vi "Write Power FIFO Direct Dispatch.vi"(6 "FIFO Timestamps":T2, 8 "error in (no error)":errorcluster, 9 "Timeout (ms)":i32=100, 10 "Power Waveform In":T1, 11 "CIFTag in":refnum<class "CIFChannels.lvclass">) -> (0 "error out":errorcluster, 1 "timed out?":bool, 2 "Power Waveform Out":T1, 3 "CIFTag out":refnum<class "CIF_NIChn_Fifo_Power_DVR.lvclass">)   [LabVIEW 2021, in "CIF_NIChn_Fifo_Power_DVR.lvclass"]
uses:
  CIF_NIChn_Fifo_Power_DVR.lvclass
  D:/dev/CIF-LVCore/src/Channels/CIFChannels/CIFChannels.lvclass
  D:/dev/CIF-LVCore/src/Channels/CIF_NIChn/NIChn/CIF_NIChn.lvclass
  CIFChannels/CIFChannels.lvclass
  ChannelCommon/typedef/TimeStamps.ctl
  ChannelCommon/typedef/Datatype Power Waveform.ctl
  CIF_NIChn_Fifo_Power_DVR.lvclass/CIF_NIChn_Fifo_Power_DVR.ctl
  ChannelCommon/CIFFIFO/CIFfifo.lvclass/CIFfifo.ctl
  NIChn/CIF_NIChn.lvclass/CIF_NIChn.ctl
  ChannelCommon/Utilities/Get Waveform DVRs.vi
  <vilib>/CIFChannels/Top Level/Write Variable Length U8 Array.vi
  NIChn/Accessors/Read CIF Channel.vi
  NIChn/Accessors/Write CIF Channel.vi
  SubVIs/Flatten.vi
  ChannelCommon/CIFFIFO/Accessors/Read Length.vi
  <vilib>/CIFChannels/SubVIs/Get dll Path.vi
  ChannelCommon/CIFFIFO/Utilities/Update Header.vi
  ChannelCommon/CIFFIFO/Flatten/DVR Flatten.vi
  ChannelCommon/CIFFIFO/Accessors/Write T0.vi
  ChannelCommon/CIFFIFO/Accessors/Write T_Out.vi
  ChannelCommon/CIFFIFO/Accessors/Write ClockID.vi
  ChannelCommon/Utilities/Flatten Header.vi
  ChannelCommon/CIFFIFO/Flatten/DVR Flatten.vi/6fdbece9-bad6-4a8e-9bf7-fe1528478dd6.vi
  ChannelCommon/CIFFIFO/Accessors/Write Payload Length.vi
  ChannelCommon/CIFFIFO/Accessors/Read Header.vi
  CIFCore/Common/Utilities/Add Error.vi
  ChannelCommon/CIFFIFO/Flatten/DVR Flatten.vi/6fdbece9-bad6-4a8e-9bf7-fe1528478dd6.vi/c28b0ead-42ad-4072-80a2-aca7f2bd7ce3.vi
  CIFCore/Common/Utilities/Append Error Location.vi
  ChannelCommon/Utilities/Update Time.vi
  ChannelCommon/ChannelCommon.lvlib
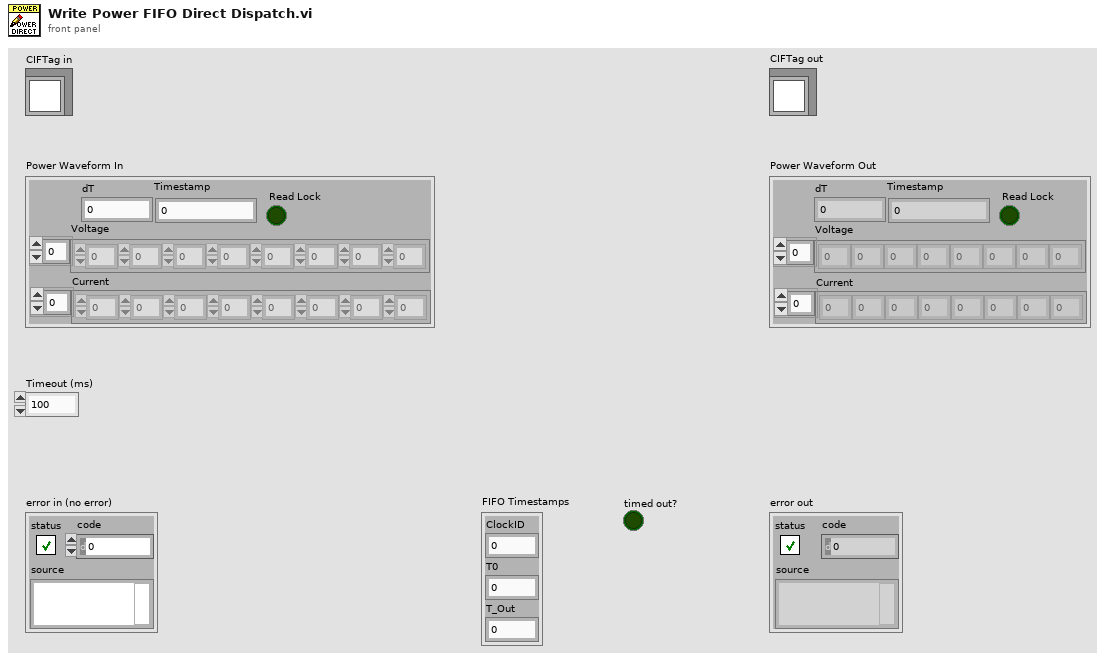
[diagram p1: front panel]
types:
  T1 = typedef "ChannelCommon.lvlib/Datatype Power Waveform.ctl" = cluster{"Voltage":dbl[], "Current":dbl[], "dT":dbl, "Timestamp":u64, "Read Lock":bool}
  T2 = typedef "ChannelCommon.lvlib/TimeStamps.ctl" = cluster{"ClockID":u8, "T0":u64, "T_Out":u64}
  T3 = typedef "ChannelCommon.lvlib/Datatype Waveform.ctl" = cluster{"measurement":dbl[], "dT":dbl, "Timestamp":u64, "Read Lock":bool}
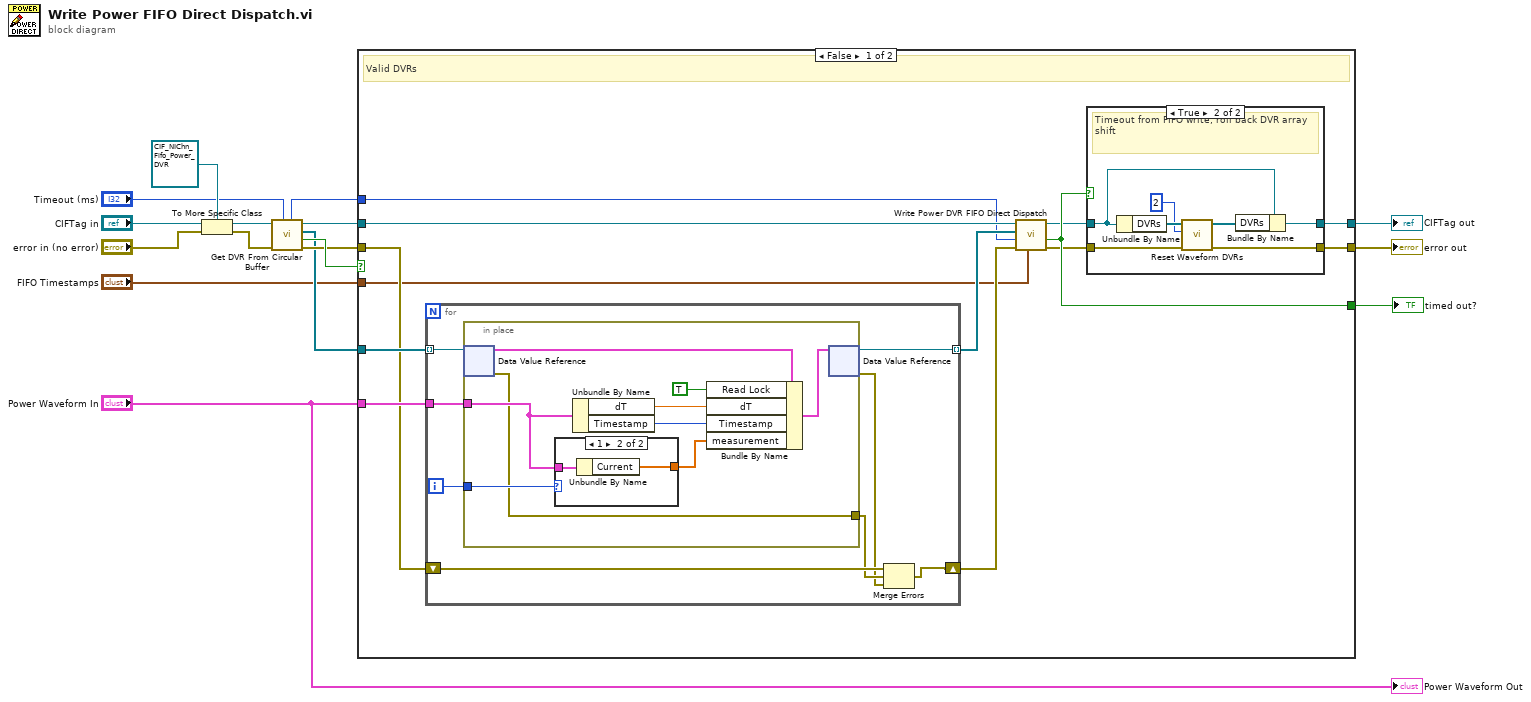
[diagram p0: block diagram]
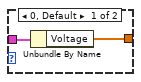
[diagram p3: hidden frame]
diagram:
  n1 = To More Specific Class(target class=refnum<class "CIF_NIChn_Fifo_Power_DVR.lvclass"> refnum ("CIFTag in"), reference="CIFTag in", error in="error in (no error)") -> (specific class reference=w13:refnum<class "CIF_NIChn_Fifo_Power_DVR.lvclass">, error out=w12:errorcluster)
  n2 = call "Get DVR From Circular Buffer.vi"("Timeout in (ms)"="Timeout (ms)", "error in (no error)"=w12, "CIF_NIChn_Fifo_Power_DVR in"=w13) -> ("error out"=w10:errorcluster, "Timeout"=w11:bool, "DVRs"=w8:refnum<data-value>[], "CIF_NIChn_Fifo_Power_DVR out"=w9:refnum<class "CIF_NIChn_Fifo_Power_DVR.lvclass">, "Remaining timeout (ms)"=w1:i32)  [unwired: 4 in]
  n3 = case shown="False" w11 {
    selector: w11 -> [_ w60]
    tunnel: w10 -> [w26 w61]
    tunnel: w9 -> [w29 w62]
    tunnel: w8 -> [w28 _]
    tunnel: [w19 w62] -> w7
    tunnel: [w21 w60] -> w6
    tunnel: [w17 w61] -> w5
    tunnel: "Power Waveform In" -> [w27 _]
    tunnel: "FIFO Timestamps" -> [w23 _]
    tunnel: w1 -> [w22 _]
    frame False {
      # "Valid DVRs"
      n4 = for {
        tunnel: w28 -> [w46] mode=indexing
        tunnel: w27 -> [w45]
        tunnel: [w43] -> w24 mode=indexing
        shift-right: [w39] -> w25
        shift-left: w26 -> [w42]
        i -> [w44]
        n5 = in-place {
          in-place-border: w45 -> [w51]
          in-place-border: w44 -> [w52]
          in-place-border: [w48] -> w41
          n6 = in-place-dvr #1(w46) -> (w55:T3, w48:errorcluster)
          n7 = case shown="1" w52 {
            tunnel: w51 -> [w57 w59]
            tunnel: [w56 w58] -> w50
            frame 0, Default {
              n8 = Unbundle By Name(w57) -> ("Voltage"=w56:dbl[])
            }
            frame 1 {
              n9 = Unbundle By Name(w59) -> ("Current"=w58:dbl[])
            }
          }
          n10 = Unbundle By Name(w51) -> ("dT"=w54:dbl, "Timestamp"=w53:u64)
          n11 = Bundle By Name(cluster=w55, "Read Lock"=TRUE, "dT"=w54, "Timestamp"=w53, "measurement"=w50) -> (w49:T3)
          n12 = in-place-dvr #1(w49) -> (w43:refnum<data-value>, w40:errorcluster)
        }
        n13 = Merge Errors(w42, w41, w40) -> (w39:errorcluster)
      }
      n14 = call "Write Power DVR FIFO Direct Dispatch.vi"("FIFO Timestamps"=w23, "error in (no error)"=w25, "Timeout (ms)"=w22, "Data In"=w24, "CIFTag in"=w29) -> ("error out"=w18:errorcluster, "timed out?"=w21:bool, "CIFTag out"=w20:refnum<class "CIF_NIChn_Fifo_Power_DVR.lvclass">)  [unwired: 3 in, 1 out]
      n15 = case shown="True" w21 {
        tunnel: w20 -> [w31 w38]
        tunnel: [w31 w37] -> w19
        tunnel: w18 -> [w30 w36]
        tunnel: [w30 w35] -> w17
        frame False {
        }
        frame True {
          # "Timeout from FIFO write, roll back DVR array shift"
          n16 = Unbundle By Name(w38) -> ("DVRs"=w33:refnum<data-value>[])
          n17 = call "Reset Waveform DVRs.vi"("error in (no error)"=w36, "Number of Waveforms"=2, "DVR Circular Buffer in"=w33) -> ("error out"=w35:errorcluster, "DVR Circular Buffer out"=w34:refnum<data-value>[])  [unwired: 7 in]
          n18 = Bundle By Name(cluster=w38, "DVRs"=w34) -> (w37:refnum<class "CIF_NIChn_Fifo_Power_DVR.lvclass">)
        }
      }
    }
    frame True {
      # "Timeout getting unlocked DVRs"
    }
  }
  "error out" <- w5
  "CIFTag out" <- w7
  "timed out?" <- w6
  "Power Waveform Out" <- "Power Waveform In"
